vi "Write_var.vi"() -> ()   [LabVIEW 2014]
uses:
  Global_var.vi
panel:
  in  "停止 2":bool
  in  "停止":bool
  out "Global_Planner_Recyle 2":dbl
  in  "Global_Planner_Recyle":dbl
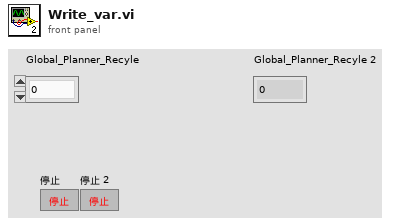
[diagram p1: front panel]
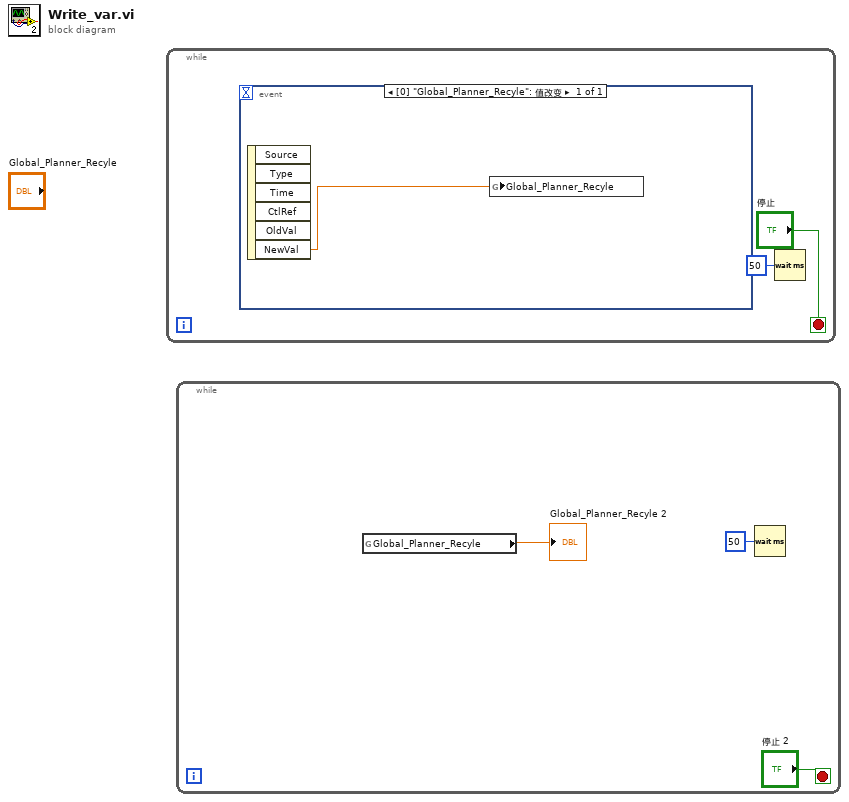
[diagram p0: block diagram]
diagram:
  n1 = while {
    stop <- "停止" stop-if-true
    n2 = event shown="[0] \"Global_Planner_Recyle\": 值改变" {
      selector: _ -> [_]
      dyn-events: _ -> [_]
      timeout: _ -> [_]
      event "Global_Planner_Recyle": Value Change {
        n3 = event-data() -> ("NewVal"=w3:dbl)  [unwired: 1 in, 5 out]
        n4 = global write "Global_var.vi" "Global_Planner_Recyle"(w3) -> ()
      }
    }
    n5 = Wait (ms)(milliseconds to wait=u32 50 ("等待时间（毫秒）")) -> ()  [unwired: 1 out]
  }
  n6 = while {
    stop <- "停止 2" stop-if-true
    n7 = global read "Global_var.vi" "Global_Planner_Recyle"() -> (→"Global_Planner_Recyle 2":dbl)
    n8 = Wait (ms)(milliseconds to wait=u32 50 ("等待时间（毫秒）")) -> ()  [unwired: 1 out]
  }
